vi "PGCalcWaits.vi"(8 "Extra Waits":i32, 9 "Cycle time\n(ms)":i32=3 min=0 step=1, 10 "BIN":u16(ring) items=["1x1", "2x2", "4x4"], 11 "MODE":u16(ring) items=["Normal", "DIF"]) -> (3 "Wait":i32)   [LabVIEW 2018]
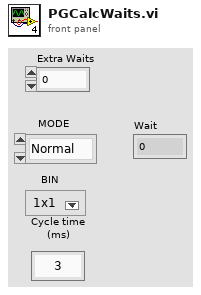
[diagram p1: front panel]
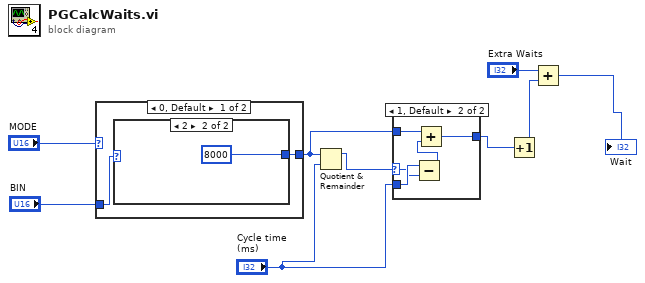
[diagram p0: block diagram]
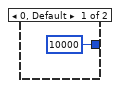
[diagram p3: hidden frame]
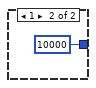
[diagram p4: hidden frame]
diagram:
  n1 = case shown="0, Default" "MODE" {
    tunnel: "BIN" -> [w11 _]
    tunnel: [w10 10000] -> w6
    frame 0, Default {
      n2 = case shown="2" w11 {
        tunnel: [10000 8000] -> w10
        frame 0, Default {
        }
        frame 2 {
        }
      }
    }
    frame 1 {
    }
  }
  n3 = Quotient & Remainder(x=w6, y="Cycle time\n(ms)") -> (x-y*floor(x/y)=w7:i32)  [unwired: 1 out]
  n4 = case shown="1, Default" w7 {
    selector: w7 -> [_ w17]
    tunnel: w6 -> [w15 w19]
    tunnel: "Cycle time\n(ms)" -> [_ w18]
    tunnel: [w15 w16] -> w4
    frame 0 {
    }
    frame 1, Default {
      n5 = Subtract(x=w18, y=w17) -> (x-y=w20:i32)
      n6 = Add(x=w19, y=w20) -> (x+y=w16:i32)
    }
  }
  n7 = Increment(x=w4) -> (x+1=w3:i32)
  n8 = Add(x="Extra Waits", y=w3) -> (x+y=→"Wait":i32)
